vi "Id2TypeColor.vi"(10 "Acc N":i32[](array[numeric]), 11 "PreIds":i32[](array[numeric])) -> (2 "Colors":u32[](array[numeric]), 3 "Pre Types":T1[](array[typedef]))   [LabVIEW 2013]
uses:
  Controls/Type of Neuron.ctl
  Controls/Neuron Info.ctl
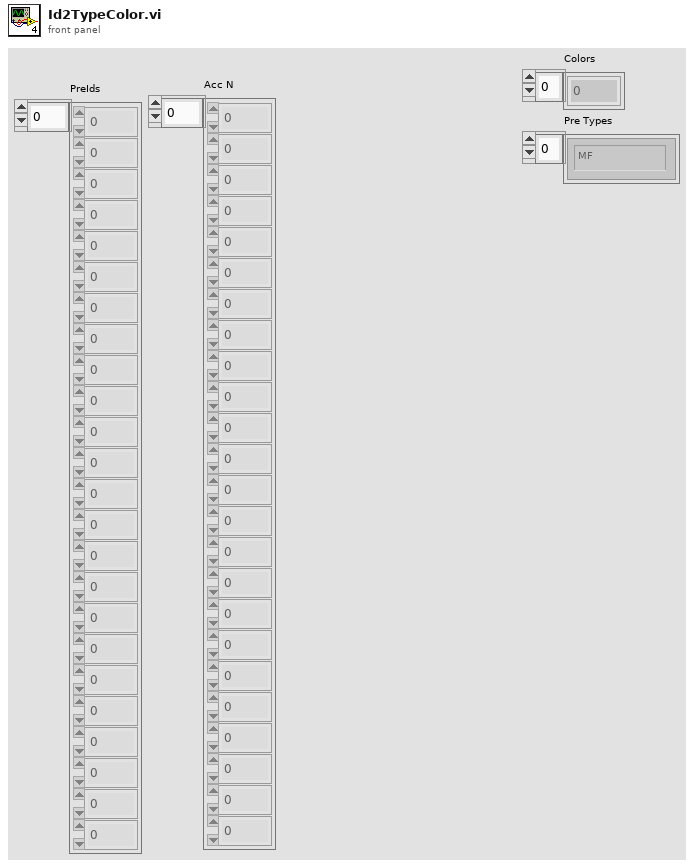
[diagram p1: front panel]
types:
  T1 = typedef "Type of Neuron.ctl" = enum16{"MF", "BA", "GO", "GC", "PC", "LU", "Glia (Dummy)"}
  T2 = typedef "Neuron Info.ctl" = cluster{"N":i32, "Radius":dbl, "Type":T1, "Color":u32}[]
  T3 = cluster{"N":i32, "Radius":dbl, "Type":T1, "Color":u32}
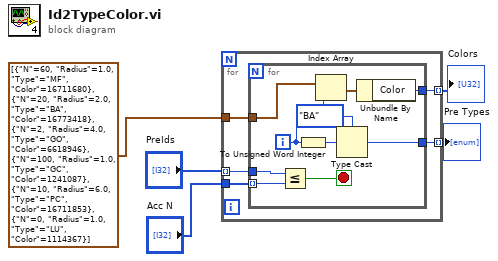
[diagram p0: block diagram]
diagram:
  n1 = for {
    tunnel: "PreIds" -> [w10] mode=indexing
    tunnel: [w9] -> w5 mode=indexing
    tunnel: T2 [{"N"=60, "Radius"=1.0, "Type"=enum."MF", "Color"=16711680}, {"N"=20, "Radius"=2.0, "Type"=enum."BA", "Color"=16773418}, {"N"=2, "Radius"=4.0, "Type"=enum."GO", "Color"=6618946}, {"N"=100, "Radius"=1.0, "Type"=enum."GC", "Color"=1241087}, {"N"=10, "Radius"=6.0, "Type"=enum."PC", "Color"=16711853}, {"N"=0, "Radius"=1.0, "Type"=enum."LU", "Color"=1114367}] ("Neurons Info") -> [w8]
    tunnel: [w7] -> w2 mode=indexing
    tunnel: "Acc N" -> [w6]
    n2 = for {
      tunnel: w10 -> [w20]
      tunnel: [w16] -> w9
      tunnel: w8 -> [w15]
      tunnel: [w12] -> w7
      tunnel: w6 -> [w11] mode=indexing
      i -> [w14]
      stop <- w19 stop-if-true
      n3 = Less Or Equal?(x=w20, y=w11) -> (x <= y?=w19:bool)
      n4 = To Unsigned Word Integer(number=w14) -> (unsigned 16bit integer=w18:u16)
      n5 = Index Array(array=w15, index=w14) -> (element=w13:T3)
      n6 = Type Cast(type=Type_of_Neuron."BA" ("Type of Neuron"), x=w18) -> (*(type *) &x=w16:T1)
      n7 = Unbundle By Name(w13) -> ("Color"=w12:u32)
    }
  }
  "Pre Types" <- w5
  "Colors" <- w2
